vi "Destroy.vi"(8 "error in (no error)":errorcluster, 11 "JKI SM in":refnum<class "JKI SM.lvclass">) -> (0 "error out":errorcluster)   [LabVIEW 2020, in "JKI State Machine API.lvlib" / "JKI SM.lvclass"]
uses:
  JKI SM.lvclass
  JKI SM.lvclass/JKI SM.ctl
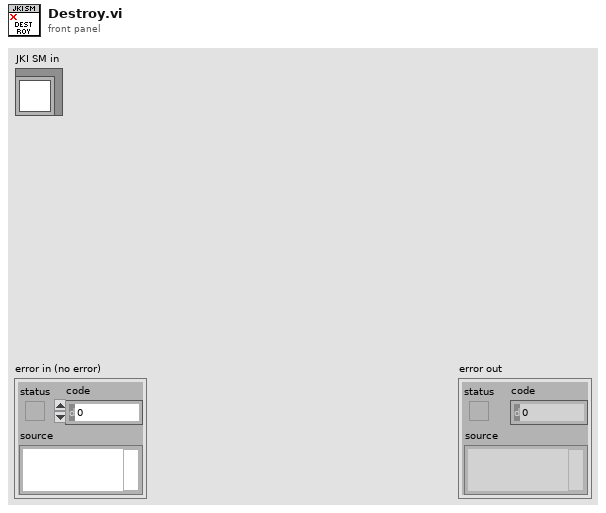
[diagram p1: front panel]
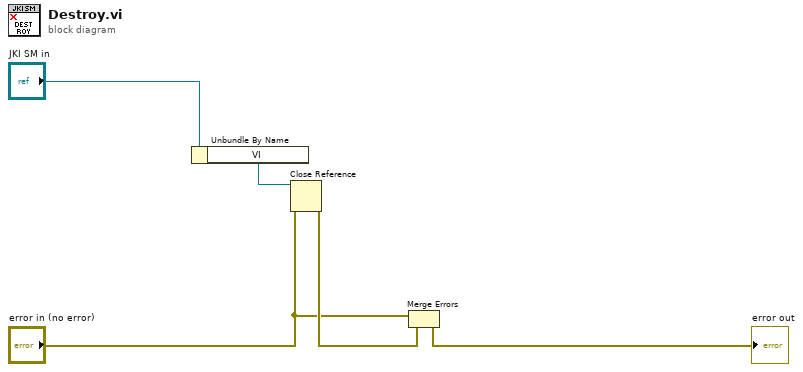
[diagram p0: block diagram]
diagram:
  n1 = Unbundle By Name("JKI SM in") -> ("VI"=w4:refnum<vi>)
  n2 = Close Reference(reference=w4, error in (no error)="error in (no error)") -> (error out=w3:errorcluster)
  n3 = Merge Errors("error in (no error)", w3) -> (→"error out":errorcluster)
